vi "CPP-Equation.vi"(4 "Scan Period":dbl format="%.2f", 5 "Previous Scan Value":dbl format="%.2f", 6 "Present scan array":dbl[](array[numeric]) format="%.2f", 7 "Value to Output":dbl format="%.2f", 8 "Ch Description":T1={"Ch Name"="", "Type"="Help", "Function"=enum."Analogue Input", "Ch State"=enum."On", "Calibration type"="", "A"=0.0, "B"=0.0, "C"=0.0, "D"=0.0, "Comments"="", "Address"={"Main"=0, "Ch."=0, "Sub"=0, "Port Name"=""}, "String"="<<an:example:channel>>+<<another:channel>>", "Duty"=65535} {"Duty" format="%016b"; "D" format="%#_5g"; "C" format="%#_5g"; "B" format="%#_5g"; "A" format="%#_5g"}, 9 "Ch names":string[](array[string])) -> (0 "Scan comment":string, 1 "Output":dbl=nan format="%.4g", 3 "HelpText":string="Evaluates the equation (<<an:example:channel>>+<<another:channel>>) in the Blue (string) Box\n\nIf the keyword \"!NotNaN\" is in the Red (comment) box, then the previous value will be held if the equation yields NaN.")   [LabVIEW 2021]
doc: "Wrapper for CPP-ZerosMaintenance.vi\nChannels Names should have the format \"Tunnel#:Pressures:\" (e.g. Tunnel1:Pressures: or Tunnel3:Pressures:). A = SecondsToMonitor (intervall to determine if tunnel has been off long enough and to inspect zero drift. B = SecondsToAverage (averaging interval for transducer zeros)."
uses:
  ADAM Client/Sub VIs/ADAM Controls/Ch_description_ADAM.ctl
  ADAM Client/Sub VIs/ADAM Controls/Module_type_ADAM.ctl
  ADAM Client/Sub VIs/ADAM Controls/Function_ADAM.ctl
  ADAM Client/Sub VIs/ADAM Controls/Channel_State.ctl
  ADAM Client/Sub VIs/ADAM Controls/Calib_type_ADAM.ctl
  ADAM Client/Sub VIs/ADAM Controls/Address.ctl
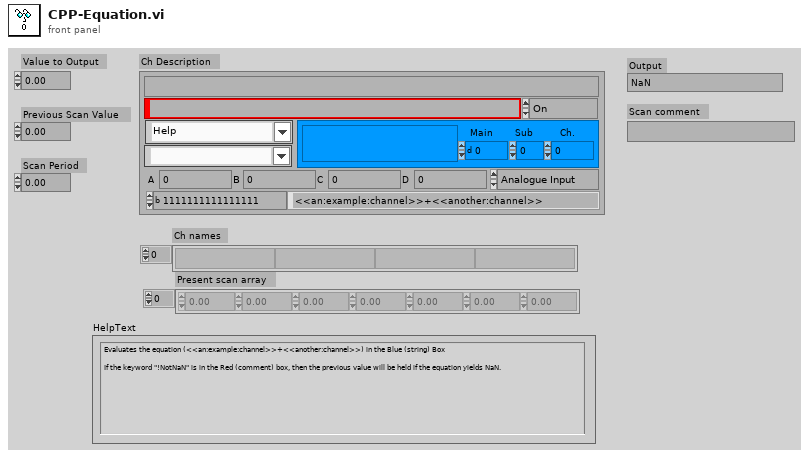
[diagram p1: front panel]
types:
  T1 = typedef "Ch_description_ADAM.ctl" = cluster{"Ch Name":string, "Type":T2, "Function":T3, "Ch State":T4, "Calibration type":T5, "A":dbl, "B":dbl, "C":dbl, "D":dbl, "Comments":string, "Address":T6, "String":string, "Duty":u16}
  T2 = typedef "Module_type_ADAM.ctl" = string
  T3 = typedef "Function_ADAM.ctl" = enum16{"Analogue Input", "Digital Input", "Event counter", "Event rate", "Analogue Output", "Digital Output", "Relay Output"}
  T4 = typedef "Channel_State.ctl" = enum16{"On", "Off", "Always On", "Always Off"}
  T5 = typedef "Calib_type_ADAM.ctl" = string
  T6 = typedef "Address.ctl" = cluster{"Main":i32, "Ch.":i32, "Sub":i32, "Port Name":string}
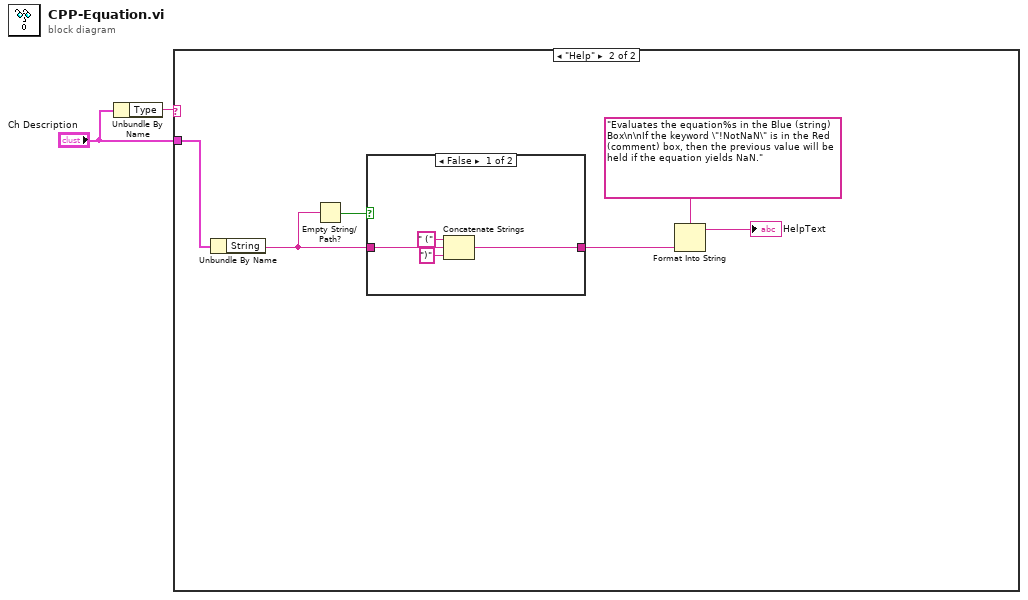
[diagram p0: block diagram]
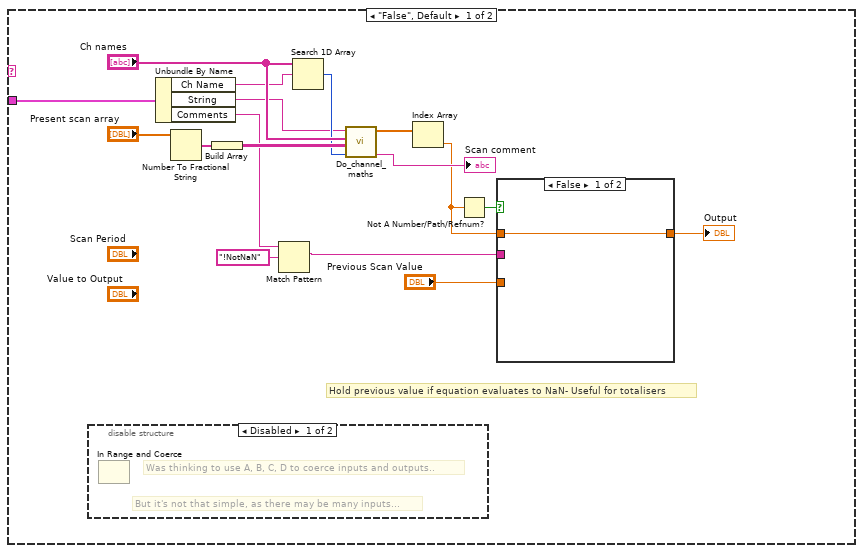
[diagram p2: hidden frame]
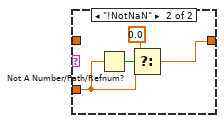
[diagram p4: hidden frame]
diagram:
  n1 = Unbundle By Name("Ch Description") -> ("Type"=w1:T2)
  n2 = case shown="\"Help\"" w1 {
    tunnel: "Ch Description" -> [w19 w35]
    frame "False", Default {
      # "Hold previous value if equation evaluates to NaN- Useful for totalisers"
      n3 = disable-structure shown="Disabled" {
        frame Disabled {
          # "But it's not that simple, as there may be many inputs..."
          # "Was thinking to use A, B, C, D to coerce inputs and outputs.."
          n4 = In Range and Coerce() -> ()  [unwired: 3 in, 2 out]
        }
        frame Enabled {
        }
      }
      n5 = Unbundle By Name(w19) -> ("Ch Name"=w12:string, "String"=w13:string, "Comments"=w9:string)
      n6 = Number To Fractional String(number="Present scan array") -> (F-format string=w18:string[])  [unwired: 3 in]
      n7 = Build Array(w18) -> (w17:string[][])
      n8 = Match Pattern(string=w9, regular expression="!NotNaN") -> (match substring=w4:string)  [unwired: 1 in, 3 out]
      n9 = Search 1D Array(1D array="Ch names", element=w12) -> (index of element=w14:i32)  [unwired: 1 in]
      n10 = call "Do_channel_maths.vi"("Output Index"=w14, "Channel Values In"=w17, "Channel Names"="Ch names", "Maths Equation"=w13) -> ("Error String"=→"Scan comment":string, "Results"=w11:dbl[])  [unwired: 1 in, 1 out]
      n11 = Index Array(array=w11) -> (element=w6:dbl)  [unwired: 1 in]
      n12 = Not A Number/Path/Refnum?(number/path/refnum=w6) -> (NaN/Path/Refnum?=w7:bool)
      n13 = case shown="False" w7 {
        tunnel: [w20 w23] -> w5
        tunnel: w6 -> [w20 w21]
        tunnel: w4 -> [_ w24]
        tunnel: "Previous Scan Value" -> [_ w22]
        frame False {
        }
        frame True {
          n14 = case shown="\"False\", Default" w24 {
            tunnel: [w25 w27] -> w23
            tunnel: w22 -> [_ w28]
            tunnel: w21 -> [w25 _]
            frame "False", Default {
            }
            frame "!NotNaN" {
              n15 = Not A Number/Path/Refnum?(number/path/refnum=w28) -> (NaN/Path/Refnum?=w29:bool)
              n16 = Select(t=0.0, s=w29, f=w28) -> (s? t:f=w27:dbl)
            }
          }
        }
      }
      "Output" <- w5
    }
    frame "Help" {
      n17 = Unbundle By Name(w35) -> ("String"=w31:string)
      n18 = Empty String/Path?(string/path=w31) -> (empty?=w32:bool)
      n19 = case shown="False" w32 {
        tunnel: [w38 w40] -> w33
        tunnel: w31 -> [w39 w40]
        frame False {
          n20 = Concatenate Strings(" (" ("string"), w39, ")" ("string")) -> (w38:string)
        }
        frame True {
        }
      }
      n21 = Format Into String(format string="Evaluates the equation%s in the Blue (string) Box\n\nIf the keyword \"!NotNaN\" is in the Red (comment) box, then the previous value will be held if the equation yields NaN.", w33) -> (resulting string=→"HelpText":string)  [unwired: 2 in, 1 out]
    }
  }
